vi "1.5-MultServ.vi"   [LabVIEW 2010]
uses:
  <vilib>/Platform/TimedLoop/XDataNode/XDataNode.xnode
  <vilib>/Platform/TimedLoop/XDataNode/timing_clust.ctl
  <vilib>/Platform/TimedLoop/XDataNode/nitl_modes.ctl
  <vilib>/Platform/TimedLoop/XDataNode/wakeup.ctl
  <vilib>/rvi/DataTransferAndStorage/Container/XNode/niFpgaContainer.xnode
  <vilib>/rvi/DataTransferAndStorage/Container/Common/niFpgaTransferTypeControl.ctl
  <vilib>/rvi/FIFO/Fifo_Types/niFpgaFifoControlLogicControl.ctl
  <vilib>/rvi/DataTransferAndStorage/Container/Common/niFpgaContainerMethod.ctl
  <vilib>/rvi/DataTransferAndStorage/Container/Common/niFpgaContainerMetaDataKey.ctl
  <vilib>/rvi/DataTransferAndStorage/FIFO/niFpgaPeerToPeerStreamState.ctl
  <vilib>/rvi/FXPMathLib/FxpMul/XNode/nifxpmath_Multiplier.xnode
  <vilib>/rvi/FXPMathLib/FxpMul/subVIs/nifxpmath_Mul_SimConfig.ctl
  <vilib>/fxp/LVFixedPointQuantizationPolicyTypeDef.ctl
  <vilib>/fxp/LVFixedPointOverflowPolicyTypeDef.ctl
  1.0-Hindbrain Global.vi
  <vilib>/rvi/DataTransferAndStorage/Container/Common/niFpgaContainerExecOnDevCompGetState.vi
  <vilib>/rvi/FIFO/Fifo_Resource/nirvififoEmulationSetSize.vi
  <vilib>/rvi/DataTransferAndStorage/Container/Common/niFpgaContainerGetUniqueNameForEmu.vi
  <vilib>/rvi/interface/RandomDataEmulation/nirviRandomDataFPGAFIFO.vi
  <vilib>/rvi/interface/RandomDataEmulation/niFpgaRandomDataHandleErrors.vi
  <vilib>/rvi/eio/common/nirviEmuReportErrorAndStop.vi
  <vilib>/rvi/FXPMathLib/FxpMul/simVIs/DllFxpMulTemp_sub.vi
  <vilib>/rvi/Memory/Memory_Emulation/nirvimemoryEmulationManagerCache_GetValue.vi
  <vilib>/rvi/Memory/Memory_Emulation/nirvimemoryEmulationManagerCache_InsertValue.vi
  <vilib>/Utility/error.llb/Clear Errors.vi
  <vilib>/rvi/Memory/Memory_Emulation/nirvimemoryEmulationManagerCache_SetValue.vi
  <vilib>/Platform/TimedLoop/XDataNode/XDNodeRunTimeDep.lvlib
types:
  T1 = typedef "XDNodeRunTimeDep.lvlib/timing_clust.ctl" = cluster{"Expected End [f-1]":u64, "Actual End [f-1]":u64, "Finished Late? [f-1]":bool, "Expected End [i-1]":u64, "Actual End [i-1]":u64, "Finished Late? [i-1]":bool, "Expected Start [i]":u64, "Actual Start [i]":u64, "Expected Start [f]":u64, "Actual Start [f]":u64, "Source Name":string, "Structure Name":string, "Period":i64, "Deadline":i64, "Offset":i64, "Start":i64, "Priority":i32, "Timeout":i32, "Mode":T2, "Wakeup Reason":T3, "Error":errorcluster, "Source Type":string, "Secondary Source Type":string, "Global End Time":u64, "Global Start Time":u64, "Frame Duration":u64, "Iteration Duration":u64, "Assigned CPU":i32, "I/O Scan Engine Mode":u32}
  T2 = typedef "XDNodeRunTimeDep.lvlib/nitl_modes.ctl" = enum32{"No Change", "Process missed periods, maintain original phase", "Discard missed periods, maintain original phase", "Process missed periods, ignore original phase", "Discard missed periods, ignore original phase"}
  T3 = typedef "XDNodeRunTimeDep.lvlib/wakeup.ctl" = enum32{"Normal", "Aborted", "Asynchronous wakeup", "Timing source error", "Timed loop error", "Timeout"}
  T4 = typedef "niFpgaContainerMetaDataKey.ctl" = enum16{"FPGA FIFO", "FPGA Memory", "FPGA Register"}
  T5 = typedef "niFpgaFifoControlLogicControl.ctl" = enum16{"Slice Fabric", "Target Optimal", "Built-in"}
  T6 = typedef "niFpgaContainerMethod.ctl" = enum16{"<none>", "write", "read", "clear", "getNumberOfElementsToWrite", "getNumberOfElementsToRead", "enable", "disable", "flushAndDisable", "getStreamState", "readA", "readB", "dramWrite", "dramWriteWithByteEnables", "dramRequestData", "dramRetrieveData"}
  T7 = typedef "niFpgaTransferTypeControl.ctl" = enum16{"Target-Scoped", "Host to Target - DMA", "Target to Host - DMA", "Peer to Peer Reader", "Peer to Peer Writer", "Bidirectional"}
  T8 = typedef "niFpgaPeerToPeerStreamState.ctl" = enum16{"Unlinked", "Disabled", "Enabled", "Flushing"}
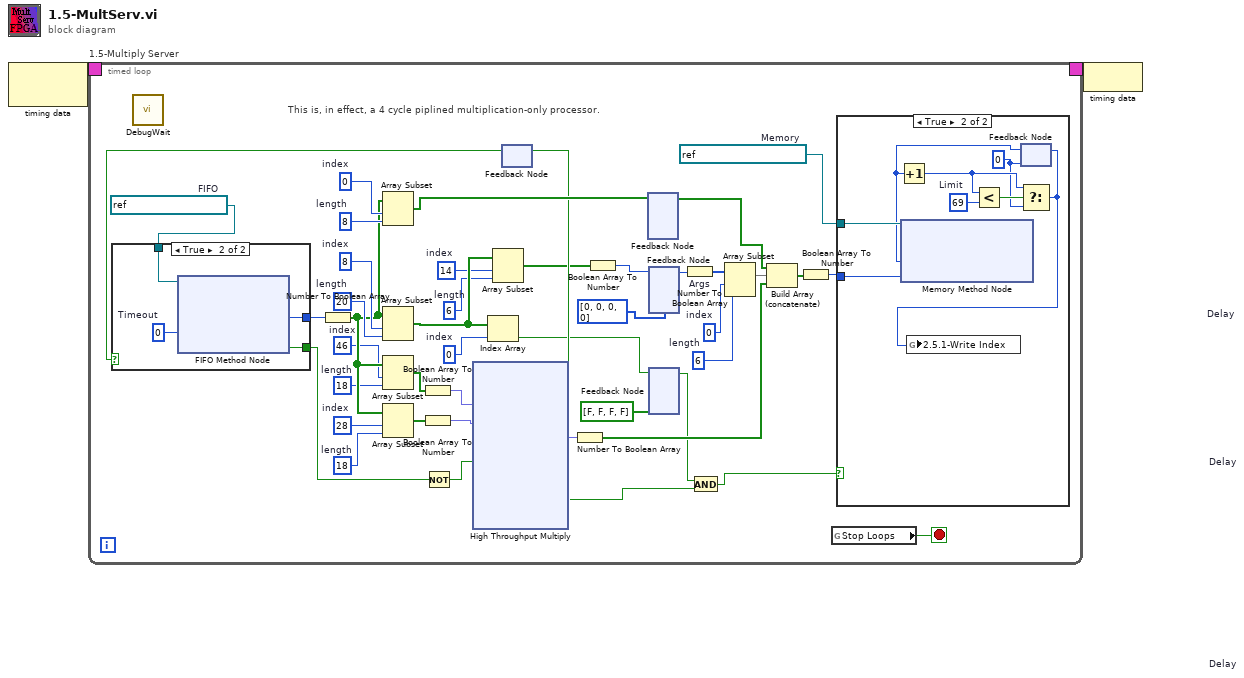
[diagram p0: block diagram]
diagram:
  n1 = node-c288() -> (w2:T1)  [unwired: 1 in]
  n2 = timed-loop "1.5-Multiply Server" {
    timing: w2 -> [_]
    timing-out: [_] -> w1
    stop <- w46 stop-if-true
    w3 = refnum<k21> "1.5.3-MultServ In"  # FIFO
    w4 = refnum<k21> "1.5.2-MultServ Out"  # Memory
    w5 = 6  # length
    w6 = 0  # index
    w13 = 6  # length
    w14 = 14  # index
    w20 = 0  # index
    w34 = 18  # length
    w35 = 46  # index
    w37 = 18  # length
    w38 = 28  # index
    w39 = 20  # length
    w40 = 8  # index
    w41 = 8  # length
    w42 = 0  # index
    # "This is, in effect, a 4 cycle piplined multiplication-only processor."
    n3 = call "DebugWait.vi"() -> ()  [unwired: 12 in]
    n4 = feedback #1() -> (w25:bool)  [unwired: 1 in]
    n5 = case shown="True" w25 {
      tunnel: w3 -> [_ w251]
      tunnel: [_ w254] -> w45
      tunnel: [_ w253] -> w43
      frame False {
      }
      frame True {
        w252 = 0  # Timeout
        n6 = xnode ("FIFO Method Node")("Timeout"=w252, "FIFO In"=w251) -> ("Element"=w253:u64, "Timed Out?"=w254:bool)  [unwired: 1 out]
      }
    }
    n7 = Number To Boolean Array(number=w43) -> (Boolean array=w36:bool[])
    n8 = Array Subset(array=w36, index=w42, length=w41) -> (w29:bool[])
    n9 = Array Subset(array=w36, index=w40, length=w39) -> (w15:bool[])
    n10 = Array Subset(array=w36, index=w35, length=w34) -> (w33:bool[])
    n11 = Array Subset(array=w36, index=w38, length=w37) -> (w32:bool[])
    n12 = Boolean Array To Number(Boolean array=w33) -> (number=w23:fxp<+/-,18,1>)
    n13 = Boolean Array To Number(Boolean array=w32) -> (number=w22:fxp<+/-,18,1>)
    n14 = Not(x=w45) -> (.not. x?=w44:bool)
    n15 = xnode "High Throughput Multiply"("x"=w23, "y"=w22, "input valid"=w44) -> ("x*y"=w31:fxp<+/-,18,1>, "output valid"=w24:bool, "ready for input"=w26:bool)  [unwired: 1 in]
    n16 = Index Array(array=w15, index=w20) -> (element=w18:bool)
    n17 = Array Subset(array=w15, index=w14, length=w13) -> (w12:bool[])
    n18 = feedback-in #1(w26) -> ()
    n19 = Number To Boolean Array(number=w31) -> (Boolean array=w28:bool[])
    n20 = Boolean Array To Number(Boolean array=w12) -> (number=w11:u8)
    n21 = feedback #2 "Delay"() -> (w21:bool[])  [unwired: 1 in]
    n22 = feedback-in #2(w29) -> ()
    n23 = feedback #3 "Delay"(u8[] [0, 0, 0, 0]) -> (w9:u8)
    n24 = feedback-in #3(w11) -> ()
    n25 = feedback #4 "Delay"(bool[] [FALSE, FALSE, FALSE, FALSE]) -> (w17:bool)
    n26 = feedback-in #4(w18) -> ()
    n27 = Number To Boolean Array "Args"(number=w9) -> (Boolean array=w8:bool[])
    n28 = And(x=w17, y=w24) -> (x .and. y?=w19:bool)
    n29 = Array Subset(array=w8, index=w6, length=w5) -> (w7:bool[])
    n30 = Build Array (concatenate)(w21, w7, w28) -> (w30:bool[])
    n31 = Boolean Array To Number(Boolean array=w30) -> (number=w27:u32)
    n32 = global read "1.0-Hindbrain Global.vi" "Stop Loops"() -> (w46:bool)
    n33 = case shown="True" w19 {
      tunnel: w4 -> [_ w54]
      tunnel: w27 -> [_ w50]
      frame False {
      }
      frame True {
        w52 = u32 69  # Limit
        w48 = u32 0
        n34 = feedback #5(w48) -> (w49:u32)
        n35 = Increment(x=w49) -> (x+1=w53:u32)
        n36 = xnode ("Memory Method Node")("Address"=w49, "Data"=w50, "Memory In"=w54) -> ()  [unwired: 1 out]
        n37 = Less?(x=w53, y=w52) -> (x < y?=w51:bool)
        n38 = Select(t=w53, s=w51, f=w48) -> (s? t:f=w47:u32)
        n39 = global write "1.0-Hindbrain Global.vi" "2.5.1-Write Index"(w47) -> ()
        n40 = feedback-in #5(w47) -> ()
      }
    }
  }
  n41 = node-c288(w1) -> ()
